vi "Emergency valve state setter.vi"(11 "Actuator Settings in":T1 {"Emergency State" items=["Closed", "Open"]; "Output Port" items=["DIDO/DO0", "DIDO/DO1", "DIDO/DO2", "DIDO/DO3", "DIDO/DO4", "DIDO/DO5", "DIDO/DO6", "DIDO/DO7", "DIDO/DO8", "DIDO/DO9", "DIDO/DO10", "DIDO/DO11", "DIDO/DO12", "DIDO/DO13", "DIDO/DO14", "DIDO/DO15", "PWM/DO0", "PWM/DO1", "PWM/DO2", "PWM/DO3", "PWM/DO4", "PWM/DO5", "PWM/DO6", "PWM/DO7"]; "Unpowered State" items=["Closed", "Opened"]}) -> (3 "Actuator Settings out":T1 {"Emergency State" items=["Closed", "Open"]; "Output Port" items=["DIDO/DO0", "DIDO/DO1", "DIDO/DO2", "DIDO/DO3", "DIDO/DO4", "DIDO/DO5", "DIDO/DO6", "DIDO/DO7", "DIDO/DO8", "DIDO/DO9", "DIDO/DO10", "DIDO/DO11", "DIDO/DO12", "DIDO/DO13", "DIDO/DO14", "DIDO/DO15", "PWM/DO0", "PWM/DO1", "PWM/DO2", "PWM/DO3", "PWM/DO4", "PWM/DO5", "PWM/DO6", "PWM/DO7"]; "Unpowered State" items=["Closed", "Opened"]})   [LabVIEW 2017]
uses:
  Controls/Manual Control FPGA.ctl
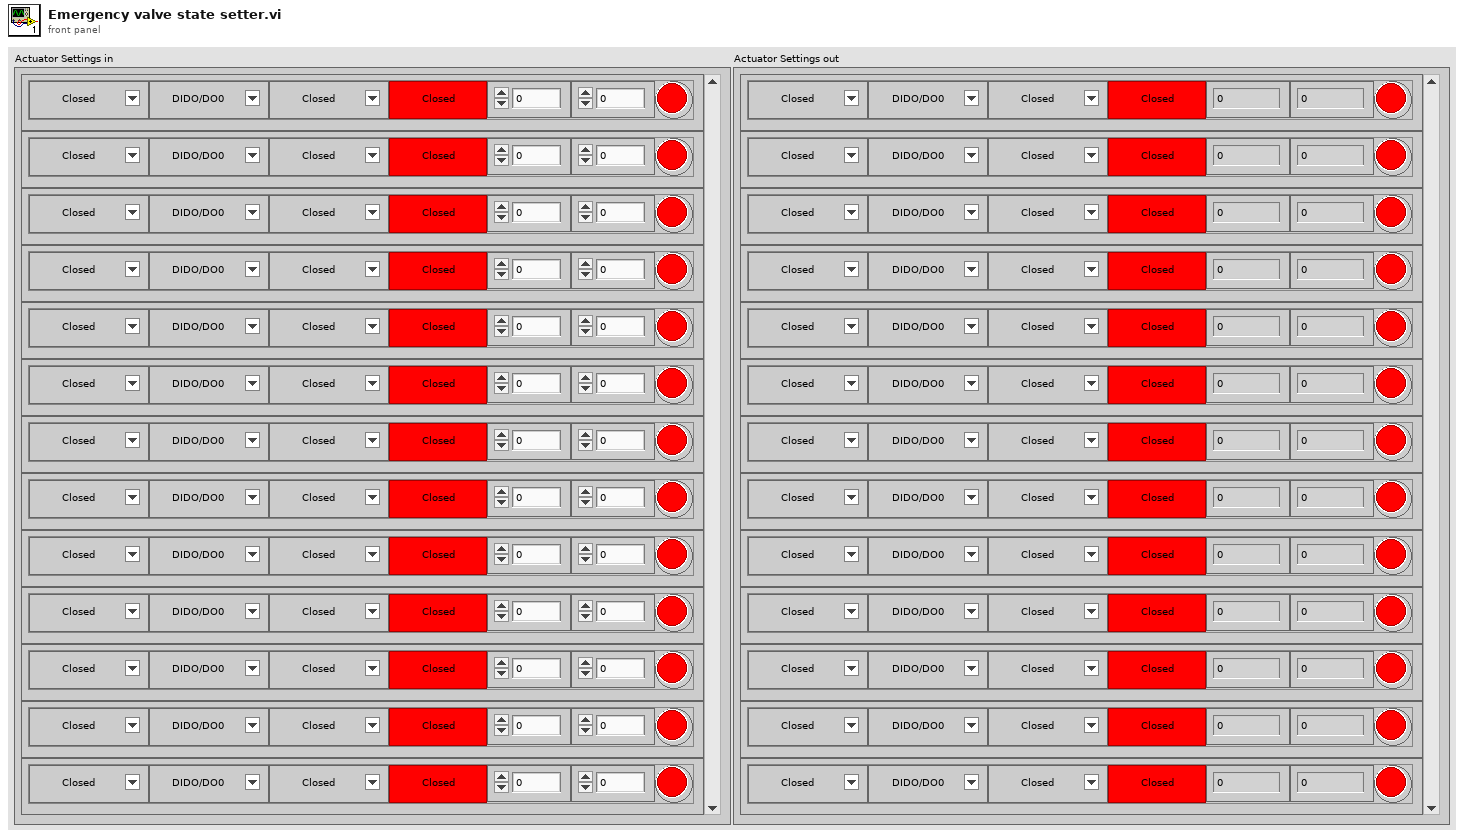
[diagram p1: front panel]
types:
  T1 = typedef "Manual Control FPGA.ctl" = cluster{"Unpowered State":i16, "Output Port":u32, "Emergency State":i16, "Blank Button":bool, "Open Time [ms]":i32, "Close Time [ms]":i32, "Active":bool}[]
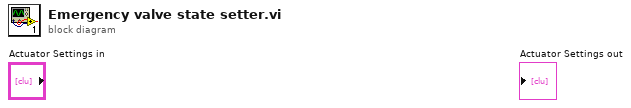
[diagram p0: block diagram]
diagram:
